vi "Save Metadata.vi"(5 "property value":variant, 7 "name":string, 8 "error in (no error)":errorcluster, 9 "channel name":string, 10 "group name":string, 11 "Logger in":refnum<class "Logger.lvclass">) -> (0 "error out":errorcluster, 1 "channel name out":string, 2 "group name out":string, 3 "Logger out":refnum<class "Logger.lvclass">)   [LabVIEW 2016, in "Logger.lvclass"]
uses:
  Logger.lvclass
  Logger.lvclass/Logger.ctl
  Read File.lvclass.vi
  Write File.lvclass.vi
  NHMFL_Core/Libraries/File/File Class/File.lvclass
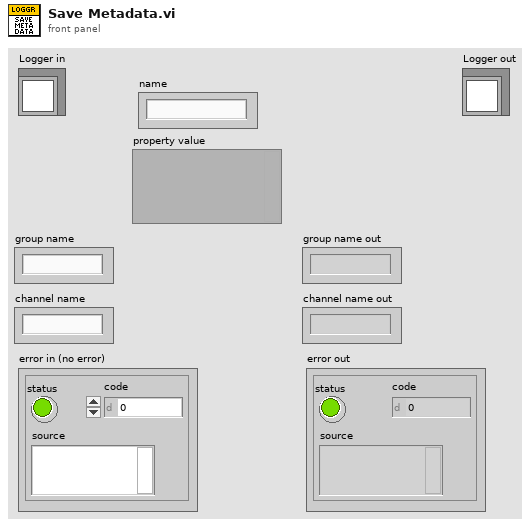
[diagram p1: front panel]
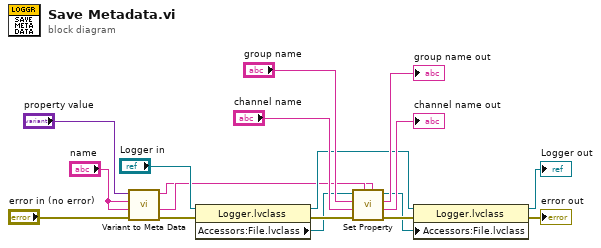
[diagram p0: block diagram]
diagram:
  n1 = call "Variant to Meta Data.vi"("Error In"="error in (no error)", "Name"="name", "key (optional)"="name", "Value"="property value") -> ("Error Out"=w1:errorcluster, "Name out"=w5:string, "Meta data"=w4:string)  [unwired: 4 in, 1 out]
  n2 = property class="Logger.lvclass"(reference="Logger in", error in=w1) -> (reference out=w10:refnum<class "Logger.lvclass">, error out=w13:errorcluster, "Accessors:File.lvclass"=w8:refnum<class "File.lvclass">)
  n3 = call-dynamic "Set Property.vi"("property value"=w4, "property name"=w5, "error in (no error)"=w13, "channel name"="channel name", "group name"="group name", "File in"=w8) -> ("error out"=w14:errorcluster, "channel name out"=→"channel name out":string, "group name out"=→"group name out":string, "File out"=w7:refnum<class "File.lvclass">)  [unwired: 2 in]
  n4 = property class="Logger.lvclass"(reference=w10, error in=w14, "Accessors:File.lvclass"=w7) -> (reference out=→"Logger out":refnum<class "Logger.lvclass">, error out=→"error out":errorcluster)
